vi "WPI_Gyro_ADXRS453_ReadSensorData.vi"(8 "error in (no error)":errorcluster, 9 "Sequence":u8, 11 "SPIDevRef in":T1) -> (0 "error out":errorcluster, 1 "Sequence Out (n-1)":u8, 2 "Sensor Data (n-1)":i16, 3 "SPIDevRef out":T1, 4 "Data Good":bool)   [LabVIEW 2015, in "FRC Gyro and Accel.lvlib"]
uses:
  FRC Gyro and Accel.lvlib
  <vilib>/Rock Robotics/WPI/SPI/WPI_SPIDevRef.ctl
  <vilib>/Rock Robotics/SystemInterfaces/spilib/spi_bus.ctl
  WPI_Gyro_ADXRS453_Commands.ctl
  WPI_Gyro_ADXRS453_Status.ctl
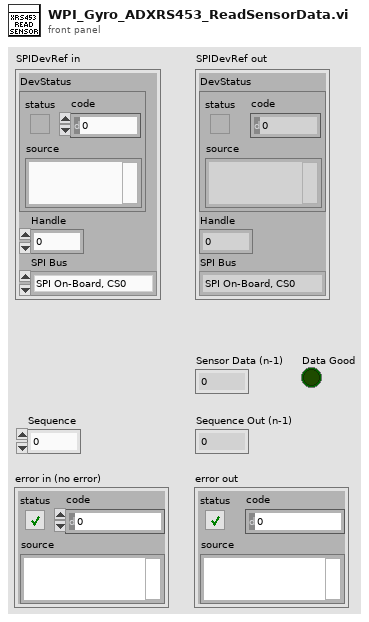
[diagram p1: front panel]
types:
  T1 = typedef "WPI_SPIDevRef.ctl" = cluster{"DevStatus":errorcluster, "Handle":i32, "SPI Bus":T2}
  T2 = typedef "spi_bus.ctl" = enum16{"SPI On-Board, CS0", "SPI On-Board, CS1", "SPI On-Board, CS2", "SPI On-Board, CS3", "SPI MXP", "Invalid"}
  T3 = typedef "FRC Gyro and Accel.lvlib/WPI_Gyro_ADXRS453_Status.ctl" = enum8{"Invalid", "Valid", "Self-Test", "Read/Write"}
  T4 = typedef "FRC Gyro and Accel.lvlib/WPI_Gyro_ADXRS453_Commands.ctl" = u8
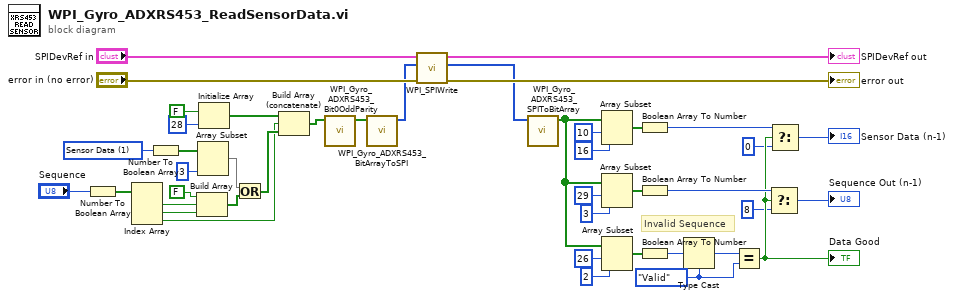
[diagram p0: block diagram]
diagram:
  w8 = WPI_Gyro_ADXRS453_Status."Valid"
  w32 = T4 1 items=["Read"=4, "Write"=2, "Sensor Data"=1]
  # "Invalid Sequence"
  n1 = Number To Boolean Array(number="Sequence") -> (Boolean array=w29:bool[])
  n2 = Index Array(array=w29) -> (element #1=w28:bool, element #2=w27:bool, element #3=w10:bool)  [unwired: 3 in]
  n3 = Number To Boolean Array(number=w32) -> (Boolean array=w33:bool[])
  n4 = Build Array(FALSE, w28, w27) -> (w25:bool[])
  n5 = Array Subset(array=w33, length=3) -> (w24:bool[])  [unwired: 1 in]
  n6 = Initialize Array(FALSE, 28 ("dimension size")) -> (w38:bool[])
  n7 = Or(x=w24, y=w25) -> (x .or. y?=w11:bool[])
  n8 = Build Array (concatenate)(w38, w10, w11) -> (w37:bool[])
  n9 = call "WPI_Gyro_ADXRS453_Bit0OddParity.vi"("Array in"=w37) -> ("Array out"=w39:bool[])  [unwired: 10 in]
  n10 = call "WPI_Gyro_ADXRS453_BitArrayToSPI.vi"("32-bit Array in"=w39) -> ("SPI Byte Array (MSB first)"=w12:u8[])  [unwired: 10 in]
  n11 = call <vilib>:"WPI_SPIWrite.vi"("error in (no error)"="error in (no error)", "Data To Send"=w12, "SPIDevRef"="SPIDevRef in") -> ("error out"=→"error out":errorcluster, "Received Data"=w18:u8[], "SPIDevRef"=→"SPIDevRef out":T1)  [unwired: 6 out]
  n12 = call "WPI_Gyro_ADXRS453_SPIToBitArray.vi"("SPI Byte Array (MSB first)"=w18) -> ("32-bit Boolean array"=w15:bool[])  [unwired: 10 in]
  n13 = Array Subset(array=w15, index=10, length=16) -> (w42:bool[])
  n14 = Array Subset(array=w15, index=29, length=3) -> (w21:bool[])
  n15 = Array Subset(array=w15, index=26, length=2) -> (w14:bool[])
  n16 = Boolean Array To Number(Boolean array=w42) -> (number=w5:i16)
  n17 = Boolean Array To Number(Boolean array=w21) -> (number=w4:u8)
  n18 = Boolean Array To Number(Boolean array=w14) -> (number=w13:u8)
  n19 = Type Cast(type=w8, x=w13) -> (*(type *) &x=w9:T3)
  n20 = Equal?(x=w9, y=w8) -> (x = y?=w3:bool)
  "Data Good" <- w3
  n21 = Select(t=w4, s=w3, f=u8 8) -> (s? t:f=→"Sequence Out (n-1)":u8)
  n22 = Select(t=w5, s=w3, f=i16 0) -> (s? t:f=→"Sensor Data (n-1)":i16)
